vi "DDT21Darray.vi"(1 "data":dynamicdata(waveform)) -> (0 "Array":dbl[](array[numeric]))   [LabVIEW 2015]
uses:
  Instance           1 19Saved   DDT21Darray .vi
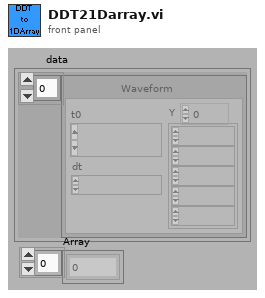
[diagram p1: front panel]
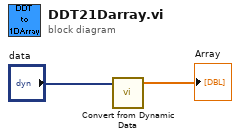
[diagram p0: block diagram]
diagram:
  n1 = call "Convert from Dynamic Data"("Dynamic Data Type"="data") -> ("Array"=→"Array":dbl[])  [unwired: 3 out]
